vi "Register0.vi"(2 "FRAC":i32, 3 "INT":i16) -> (0 "HEX0":u32 format="%08x", 1 "Reg 0":bool[](array[boolean]))   [LabVIEW 2017]
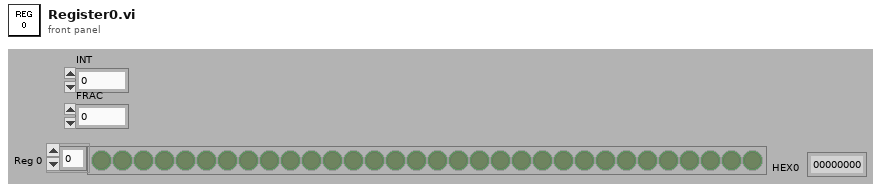
[diagram p1: front panel]
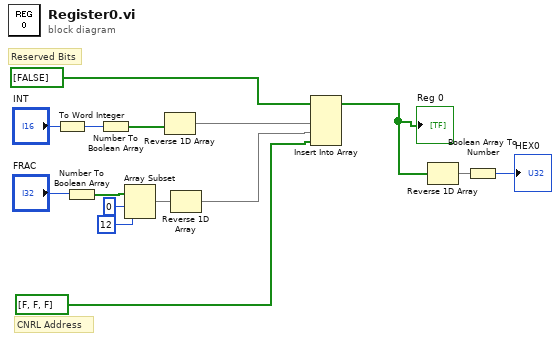
[diagram p0: block diagram]
diagram:
  # "Reserved Bits"
  # "CNRL Address"
  n1 = To Word Integer(number="INT") -> (16bit integer=w13:i16)
  n2 = Number To Boolean Array(number="FRAC") -> (Boolean array=w12:bool[])
  n3 = Number To Boolean Array(number=w13) -> (Boolean array=w11:bool[])
  n4 = Array Subset(array=w12, index=0, length=12) -> (w10:bool[])
  n5 = Reverse 1D Array(array=w11) -> (reversed array=w9:bool[])
  n6 = Reverse 1D Array(array=w10) -> (reversed array=w2:bool[])
  n7 = Insert Into Array(array=bool[] [FALSE], new element #1=w9, new element #2=w2, new element #3=bool[] [FALSE, FALSE, FALSE]) -> (w3:bool[])  [unwired: 1 in]
  "Reg 0" <- w3
  n8 = Reverse 1D Array(array=w3) -> (reversed array=w6:bool[])
  n9 = Boolean Array To Number(Boolean array=w6) -> (number=→"HEX0":u32)
